vi "RPM to rps.vi"(11 "RPM":dbl) -> (3 "rad / sec":dbl[unit])   [LabVIEW 2020]
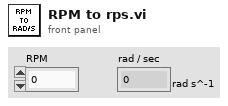
[diagram p1: front panel]
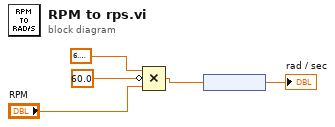
[diagram p0: block diagram]
diagram:
  n1 = Compound Arithmetic op=MULTIPLY(6.283185307179586, invert 60.0, "RPM") -> (w3:dbl)
  n2 = node(w3) -> (→"rad / sec":dbl[unit])
